vi "AOMFreqToVolt.vi"(1 "AOM freq":dbl) -> (0 "AOM voltage":dbl)   [LabVIEW 2019]
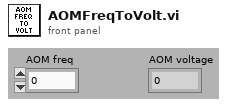
[diagram p1: front panel]
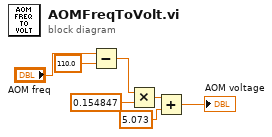
[diagram p0: block diagram]
diagram:
  n1 = Subtract(x="AOM freq", y=110.0) -> (x-y=w1:dbl)
  n2 = Multiply(x=w1, y=0.154847) -> (x*y=w5:dbl)
  n3 = Add(x=w5, y=5.073) -> (x+y=→"AOM voltage":dbl)
